vi "SUB_run_exeFile_Textv2.vi"(3 "exe filename":string) -> (0 "code":i32, 1 "standard output":string)   [LabVIEW 2011]
panel:
  out "stripped path":path
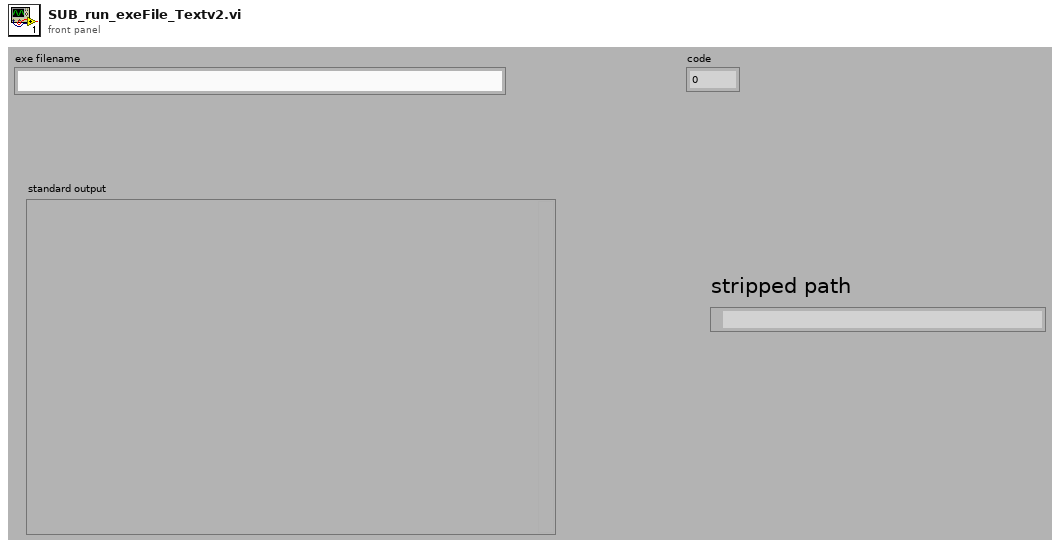
[diagram p1: front panel]
types:
  T1 = enum32{"invalid app kind", "Development System", "Run Time System", "Student Edition", "Embedded LabVIEW", "Evaluation", "Custom"}
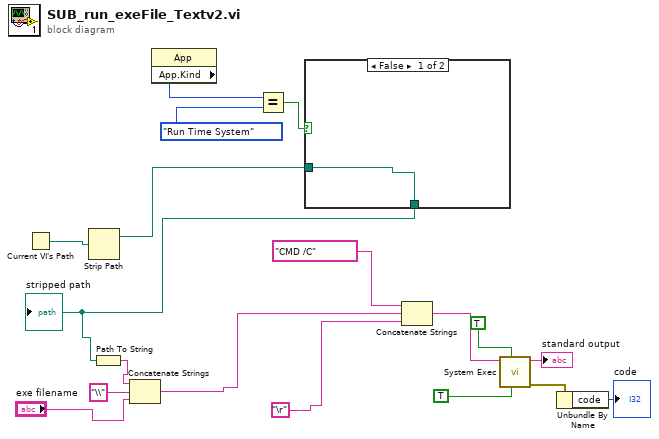
[diagram p0: block diagram]
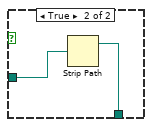
[diagram p2: hidden frame]
diagram:
  n1 = Current VI's Path() -> (path=w13:path)
  n2 = Strip Path(path=w13) -> (stripped path=w9:path)  [unwired: 1 out]
  n3 = property class="App"() -> ("App.Kind"=w10:T1)  [unwired: 2 in, 2 out]
  n4 = Equal?(x=w10, y=T1."Run Time System" ("Application:Kind")) -> (x = y?=w12:bool)
  n5 = case shown="False" w12 {
    tunnel: [w19 w21] -> w8
    tunnel: w9 -> [w19 w20]
    frame False {
    }
    frame True {
      n6 = Strip Path(path=w20) -> (stripped path=w21:path)  [unwired: 1 out]
    }
  }
  "stripped path" <- w8
  n7 = Path To String(path=w8) -> (string=w7:string)
  n8 = Concatenate Strings(w7, "\\", "exe filename") -> (w4:string)
  n9 = Concatenate Strings("CMD /C", w4, "\r") -> (w16:string)
  n10 = call <vilib>:"System Exec.vi"("run minimized? (F)"=TRUE, "wait until completion? (T)"=TRUE, "command line"=w16) -> ("error out"=w3:errorcluster, "standard output"=→"standard output":string)  [unwired: 5 in, 2 out]
  n11 = Unbundle By Name(w3) -> ("code"=→"code":i32)
